vi "Query Oscilloscope.vi"(7 "error in (no error)":errorcluster, 9 "Input Command":string="ID?", 10 "VISA resource name":refnum<visa-resource-name>) -> (0 "error out":errorcluster, 2 "read buffer":string, 3 "VISA resource out":refnum<visa-resource-name>)   [LabVIEW 2020]
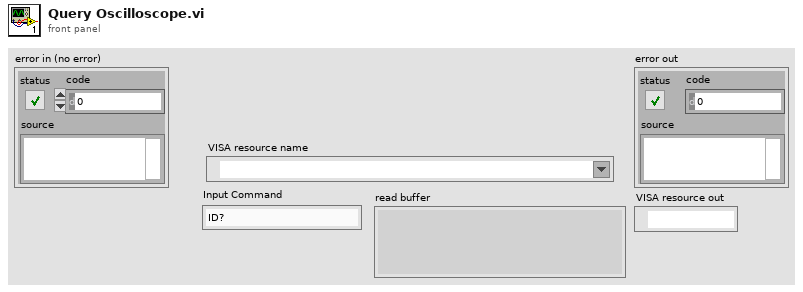
[diagram p1: front panel]
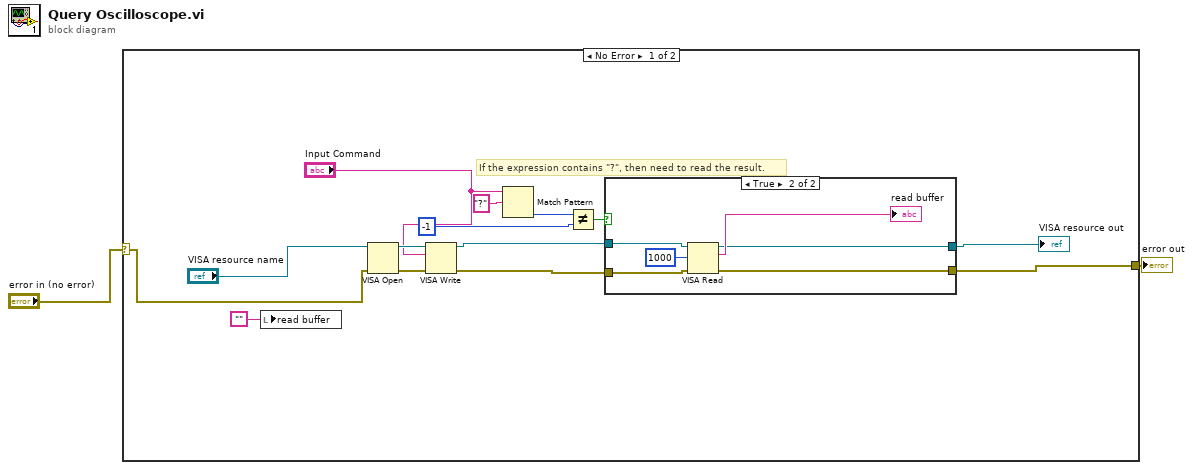
[diagram p0: block diagram]
diagram:
  n1 = case shown="No Error" "error in (no error)" {
    selector: "error in (no error)" -> [w5 w25]
    tunnel: [w4 w25] -> w2
    frame No Error {
      # "If the expression contains \"?\", then need to read the result."
      n2 = local write "read buffer"("") -> ()
      n3 = VISA Open(error in (no error)=w5, VISA resource name="VISA resource name") -> (VISA resource name=w15:refnum<visa-resource-name>, error out=w16:errorcluster)  [unwired: 3 in]
      n4 = VISA Write(VISA resource name=w15, write buffer="Input Command", error in (no error)=w16) -> (VISA resource name out=w7:refnum<visa-resource-name>, error out=w6:errorcluster)  [unwired: 1 out]
      n5 = Match Pattern(string="Input Command", regular expression="?") -> (offset past match=w12:i32)  [unwired: 1 in, 3 out]
      n6 = Not Equal?(x=w12, y=-1) -> (x != y?=w10:bool)
      n7 = case shown="True" w10 {
        tunnel: [w18 w22] -> w3
        tunnel: [w17 w21] -> w4
        tunnel: w7 -> [w18 w20]
        tunnel: w6 -> [w17 w19]
        frame False {
        }
        frame True {
          n8 = VISA Read(VISA resource name=w20, byte count=u32 1000, error in (no error)=w19) -> (VISA resource name out=w22:refnum<visa-resource-name>, read buffer=→"read buffer":string, error out=w21:errorcluster)  [unwired: 1 out]
        }
      }
      "VISA resource out" <- w3
    }
    frame Error {
    }
  }
  "error out" <- w2
